vi "Compare.vi"(9 "Headers B":refnum<class "httpHeaders.lvclass">, 11 "Headers A":refnum<class "httpHeaders.lvclass">) -> (2 "Identical?":bool)   [LabVIEW 2020, in "httpClient.lvlib" / "httpHeaders.lvclass"]
uses:
  httpHeaders.lvclass
  httpHeaders.lvclass/httpHeaders.ctl
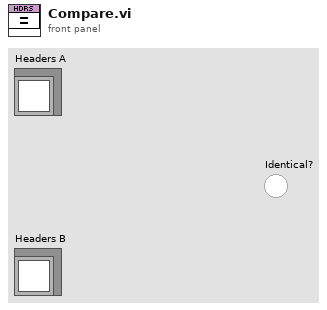
[diagram p1: front panel]
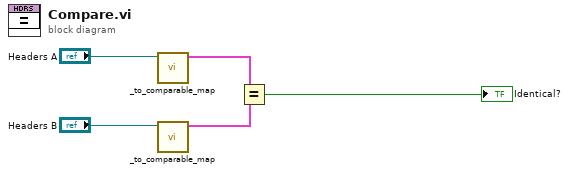
[diagram p0: block diagram]
diagram:
  n1 = call "_to_comparable_map.vi"("httpHeaders in"="Headers A") -> ("comparable headers"=w3:cluster{"header":string, "value":string}[])  [unwired: 10 in]
  n2 = call "_to_comparable_map.vi"("httpHeaders in"="Headers B") -> ("comparable headers"=w2:cluster{"header":string, "value":string}[])  [unwired: 10 in]
  n3 = Equal?(x=w3, y=w2) -> (x = y?=→"Identical?":bool)
